vi "ZLockCreate.vi"(4 "error in (no error)":errorcluster, 6 "timeout (500ms)":i32=500, 7 "app name":string) -> (0 "error out":errorcluster, 3 "ZLock out":refnum<class "ZLock.lvclass">)   [LabVIEW 2010, in "ZLock.lvclass"]
uses:
  <userlib>/bias/subvis/zlock/ZLock.lvclass
  <userlib>/bias/subvis/zlock/ZLock.lvclass/ZLock.ctl
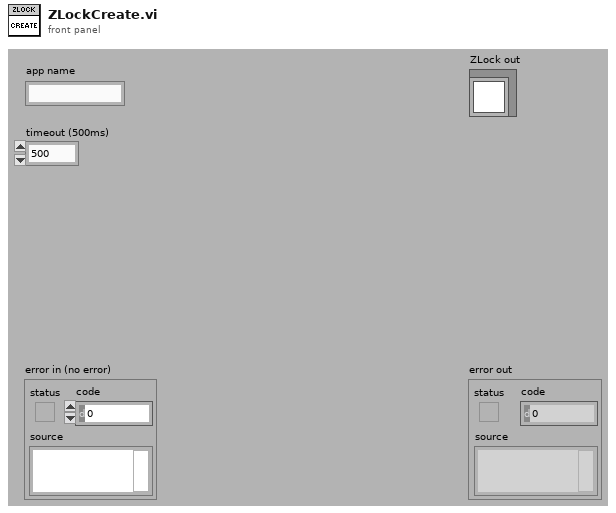
[diagram p1: front panel]
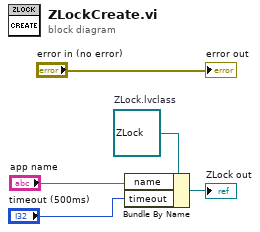
[diagram p0: block diagram]
diagram:
  w5 = refnum<class "ZLock.lvclass"> refnum  # ZLock.lvclass
  n1 = Bundle By Name(cluster=w5, "name"="app name", "timeout"="timeout (500ms)") -> (→"ZLock out":refnum<class "ZLock.lvclass">)
  "error out" <- "error in (no error)"
